vi "Boiler Points To Distance.vi"(7 "Camera Vertical FOV":dbl=34.3, 8 "Camera Height":dbl, 9 "Camera Angle":dbl, 10 "Top Tape":dbl, 11 "Bottom Tape":dbl) -> (2 "Distance (ft)":dbl)   [LabVIEW 2016]
uses:
  <vilib>/Rock Robotics/Network Tables/NT Write Number.vi
panel:
  out "Camera Rotation Offset":dbl
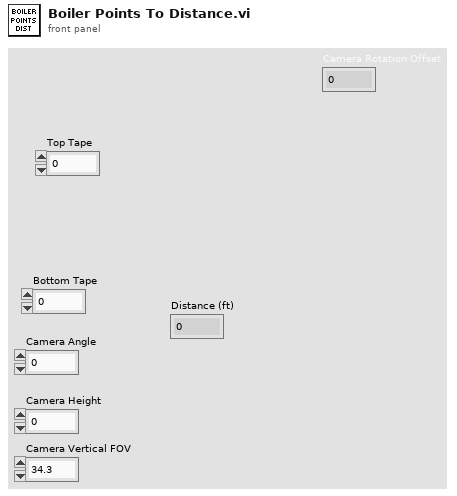
[diagram p1: front panel]
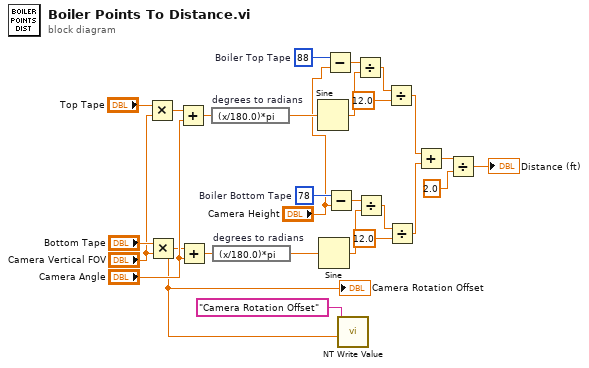
[diagram p0: block diagram]
diagram:
  w12 = 88  # Boiler Top Tape
  w27 = 78  # Boiler Bottom Tape
  n1 = Multiply(x="Top Tape", y="Camera Vertical FOV") -> (x*y=w11:dbl)
  n2 = Multiply(x="Bottom Tape", y="Camera Vertical FOV") -> (x*y=w1:dbl)
  "Camera Rotation Offset" <- w1
  n3 = Add(x=w11, y="Camera Angle") -> (x+y=w14:dbl)
  n4 = Add(x=w1, y="Camera Angle") -> (x+y=w25:dbl)
  n5 = expression code="(x/180.0)*pi" "degrees to radians"(w14) -> (w15:dbl)
  n6 = expression code="(x/180.0)*pi" "degrees to radians"(w25) -> (w24:dbl)
  n7 = Sine(x=w15) -> (sin(x)=w16:dbl)
  n8 = Sine(x=w24) -> (sin(x)=w23:dbl)
  n9 = Subtract(x=w12, y="Camera Height") -> (x-y=w13:dbl)
  n10 = Subtract(x=w27, y="Camera Height") -> (x-y=w26:dbl)
  n11 = call-poly <vilib>:"NT Write Value.vi"("Numeric"=w1, "Name"="Camera Rotation Offset") -> ()  [unwired: 9 in, 1 out]
  n12 = Divide(x=w13, y=w16) -> (x/y=w18:dbl)
  n13 = Divide(x=w26, y=w23) -> (x/y=w21:dbl)
  n14 = Divide(x=w18, y=12.0) -> (x/y=w8:dbl)
  n15 = Divide(x=w21, y=12.0) -> (x/y=w7:dbl)
  n16 = Add(x=w8, y=w7) -> (x+y=w6:dbl)
  n17 = Divide(x=w6, y=2.0) -> (x/y=→"Distance (ft)":dbl)
